vi "AutoMoveArmTimeout.vi"(7 "Action":enum16{"Lower", "Raise"}(ring), 8 "error in (no error)":errorcluster, 10 "Timeout":u32=800, 11 "CollectorArmSpeed":dbl=1.0) -> (0 "error out":errorcluster, 3 "TimedOut?":bool)   [LabVIEW 2013]
uses:
  CollectorAction.ctl
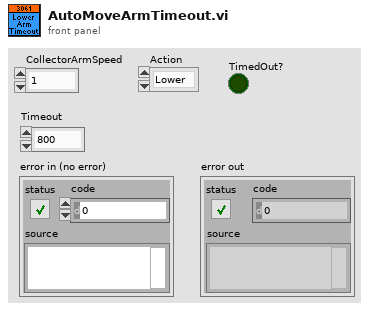
[diagram p1: front panel]
types:
  T1 = typedef "CollectorAction.ctl" = enum16{"Init", "Raise", "Lower", "Stop", "GetStatus"}
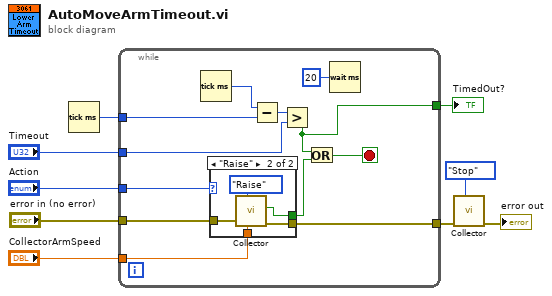
[diagram p0: block diagram]
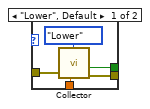
[diagram p2: hidden frame]
diagram:
  n1 = Tick Count (ms)() -> (millisecond timer value=w8:u32)
  n2 = while {
    tunnel: "error in (no error)" -> [w11]
    tunnel: [w21] -> w4
    tunnel: w8 -> [w15]
    tunnel: "CollectorArmSpeed" -> [w14]
    tunnel: [w13] -> w5
    tunnel: "Timeout" -> [w12]
    tunnel: "Action" -> [w10]
    stop <- w17 stop-if-true
    n3 = Tick Count (ms)() -> (millisecond timer value=w19:u32)
    n4 = case shown="\"Raise\"" w10 {
      tunnel: [w22 w31] -> w21
      tunnel: [w25 w27] -> w16
      tunnel: w14 -> [w24 w29]
      tunnel: w11 -> [w23 w28]
      frame "Lower", Default {
        n5 = call "Collector.vi"("MotorSpeed"=w24, "Action"=CollectorAction."Lower", "Error in"=w23) -> ("Error out"=w22:errorcluster, "Lower Triggered?"=w25:bool)  [unwired: 6 in, 1 out]
      }
      frame "Raise" {
        n6 = call "Collector.vi"("MotorSpeed"=w29, "Action"=CollectorAction."Raise", "Error in"=w28) -> ("Error out"=w31:errorcluster, "Upper Triggered?"=w27:bool)  [unwired: 6 in, 1 out]
      }
    }
    n7 = Subtract(x=w19, y=w15) -> (x-y=w20:u32)
    n8 = Greater?(x=w20, y=w12) -> (0:w13:bool)
    n9 = Or(x=w13, y=w16) -> (x .or. y?=w17:bool)
    n10 = Wait (ms)(milliseconds to wait=u32 20) -> ()  [unwired: 1 out]
  }
  "TimedOut?" <- w5
  n11 = call "Collector.vi"("Action"=CollectorAction."Stop", "Error in"=w4) -> ("Error out"=→"error out":errorcluster)  [unwired: 7 in, 2 out]
